vi "StopWatch.vi"() -> ()   [LabVIEW 2022 SP3]
panel:
  in  "?":bool
  out "Time (s)":dbl
  # "Stopwatch:"
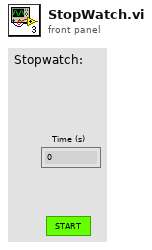
[diagram p1: front panel]
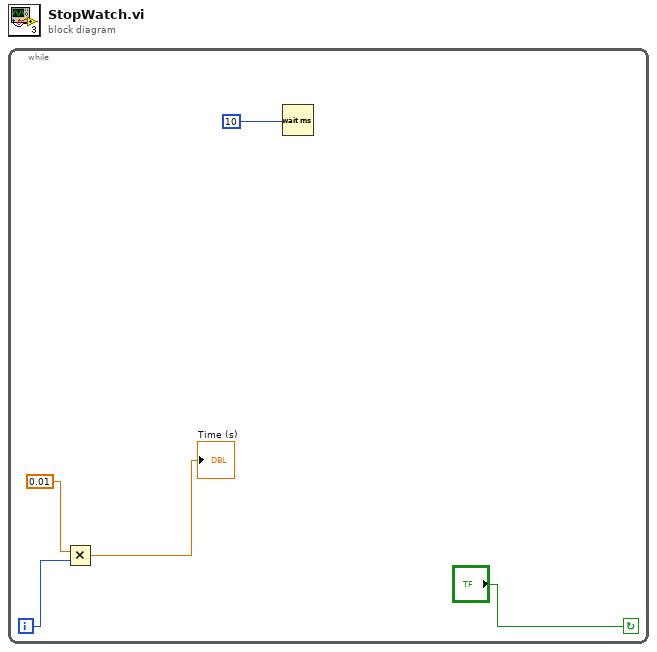
[diagram p0: block diagram]
diagram:
  n1 = while {
    i -> [w5]
    stop <- "?" continue-if-true
    n2 = Multiply(x=0.01, y=w5) -> (x*y=→"Time (s)":dbl)
    n3 = Wait (ms)(milliseconds to wait=10) -> ()  [unwired: 1 out]
  }
